vi "simulation.vi"() -> ()   [LabVIEW 2014]
uses:
  <vilib>/addons/Modulation/Digital/Support/Controls/Pack Bits Parameters.ctl
  <vilib>/addons/Modulation/Digital/General/MT Generate Bits (Galois, PN Order).vi
  <vilib>/addons/Modulation/Analog/support/mod_Set Error Source.vi
  <vilib>/addons/Modulation/Digital/Support/Common/Validators/mod_Generate Bits Validate.vi
  <vilib>/addons/Modulation/Digital/Support/Common/Validators/mod_AWGN Validate.vi
  <vilib>/addons/Modulation/Digital/Impairments/subVIs/mod_createSeeds.vi
  <vilib>/addons/Modulation/Digital/Support/Common/Validators/mod_Validate Samples Per Symbol.vi
  <vilib>/addons/Modulation/Analog/support/Validators/mod_Validate Complex Waveform.vi
  <vilib>/addons/Modulation/Analog/support/Validators/mod_WFErrorHandler.vi
  <vilib>/addons/Modulation/Digital/Support/Common/Validators/mod_Generate Filter Coefficients Validate.vi
  <vilib>/addons/Modulation/Digital/General/subVIs/mod_Generate Filter Coefficients.vi
  <vilib>/addons/Modulation/Digital/General/subVIs/mod_Generate Bits PN Sequence.vi
  <vilib>/addons/Modulation/Digital/General/MT Apply Pulse Shaping Filter (Generic).vi
  <vilib>/Analysis/1siggen.llb/Gaussian White Noise (obs 90).vi
  <vilib>/addons/Modulation/niDMT.lvlib
panel:
  out "XY Graph 2":cdb[](graph)
  in  "lpbw":dbl
  in  "nfilts":i32
  in  "noise density (dBc/Hz)":dbl=-120.0 format="%.2p"
  in  "Eb/N0 (10 dB)":dbl=10.0 format="%.2f"
  in  "bits per symbol (1)":i32=1
  out "decoded":i32
  out "iterations":i32
  out "bytes cluster":cluster{string}[](array[cluster])
  in  "type":enum16{"binary", "quadrature"}(ring)
  out "XY Graph":cdb[](graph)
  in  "total bits (128)":i32=128
  in  "stop":bool
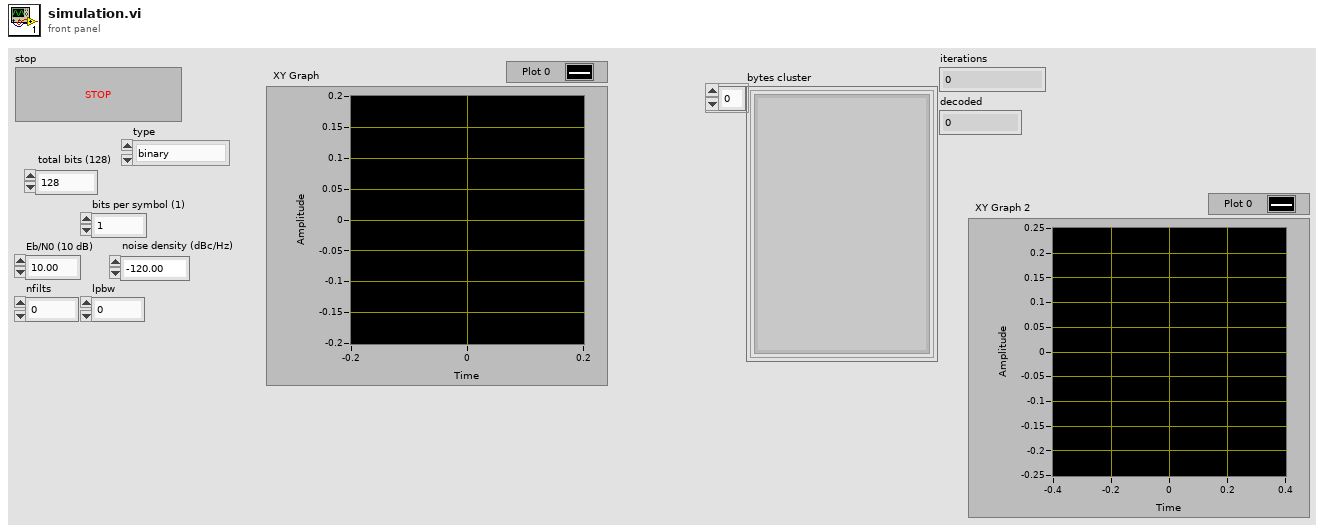
[diagram p1: front panel]
types:
  T1 = enum16{"none", "Raised Cosine", "Root Raised Cos", "Gaussian"}
  T2 = enum16{"FSK", "PSK", "QAM", "MSK", "PAM", "ASK", "CPM"}
  T3 = typedef "niDMT.lvlib/Pack Bits Parameters.ctl" = enum16{"Unsigned", "Signed"}
  T4 = typedef "niAMT.lvlib/Complex Data Waveform.ctl" = cluster{"t0":dbl, "dt":dbl, "Y":cdb[]}
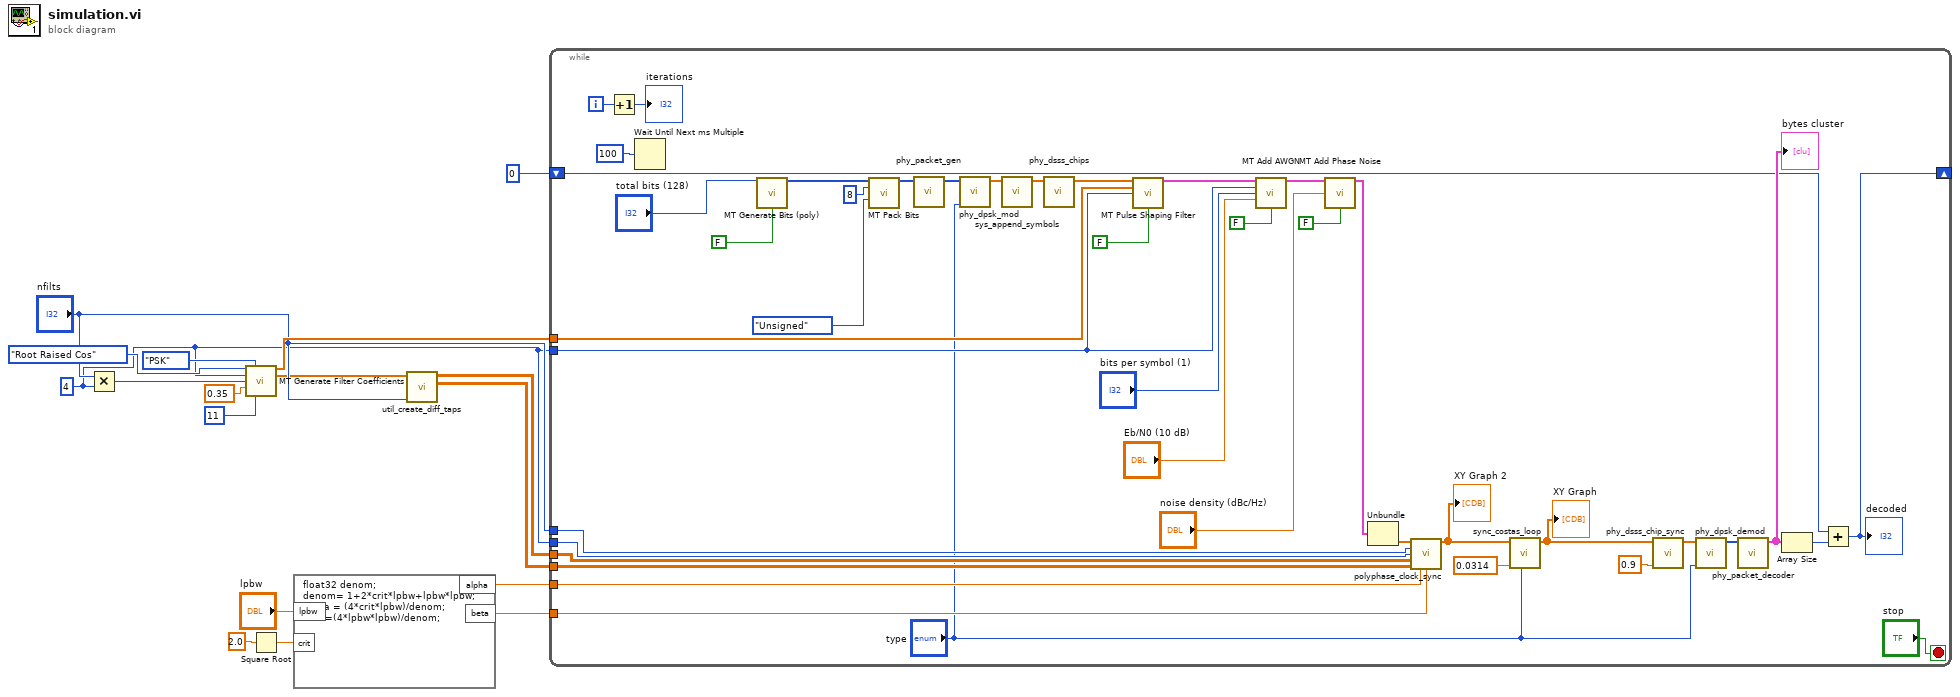
[diagram p0: block diagram]
diagram:
  w8 = 4 ("pulse shaping samples per symbol (16)")
  n1 = Multiply(x="nfilts", y=w8) -> (x*y=w1:i32)
  n2 = call <vilib>:"MT Generate Filter Coefficients.vi"("pulse shaping filter (none)"=T1."Root Raised Cos", "modulation type"=T2."PSK", "pulse shaping samples per symbol (16)"=w8, "matched samples per symbol (16)"=w1, "filter parameter"=0.35, "filter length (symbols)"=11) -> ("pulse shaping filter coefficients"=w12:dbl[], "matched filter coefficients"=w2:dbl[])  [unwired: 7 in, 1 out]
  n3 = Square Root(x=2.0) -> (sqrt(x)=w5:dbl)
  n4 = formula code="float32 denom; \ndenom= 1+2*crit*lpbw+lpbw*lpbw;\nalpha = (4*crit*lpbw)/denom;\nbeta=(4*lpbw*lpbw)/denom;"("lpbw"="lpbw", "crit"=w5) -> ("alpha"=w4:dbl, "beta"=w3:dbl)
  n5 = call "util_create_diff_taps.vi"("nfilts"="nfilts", "taps"=w2) -> ("out diff taps"=w10:dbl[][], "out taps"=w11:dbl[][])  [unwired: 7 in, 1 out]
  n6 = while {
    shift-right: [w43] -> _
    shift-left: 0 -> [w44]
    tunnel: w12 -> [w39]
    tunnel: w8 -> [w37]
    tunnel: w11 -> [w31]
    tunnel: w10 -> [w30]
    tunnel: "nfilts" -> [w29]
    tunnel: w8 -> [w28]
    tunnel: w4 -> [w27]
    tunnel: w3 -> [w26]
    i -> [w42]
    stop <- "stop" stop-if-true
    n7 = Increment(x=w42) -> (x+1=→"iterations":i32)
    n8 = Wait Until Next ms Multiple(millisecond multiple=u32 100) -> ()  [unwired: 1 out]
    n9 = call-poly <vilib>:"MT Generate Bits (poly).vi"("total bits (128)"="total bits (128)", "reset? (T)"=FALSE) -> ("output bit stream"=w55:i8[])  [unwired: 11 in, 2 out]
    n10 = call <vilib>:"MT Pack Bits.vi"("input bit stream"=w55, "bits per integer"=8, "integer format"=Pack_Bits_Parameters."Unsigned") -> ("output integers"=w52:i32[])  [unwired: 11 in, 1 out]
    n11 = call "phy_packet_gen.vi"("Input bytes"=w52) -> ("output bit stream"=w58:i8[])  [unwired: 10 in]
    n12 = call "phy_dpsk_mod.vi"("type"="type", "input bits"=w58) -> ("dpsk"=w57:cdb[])  [unwired: 8 in, 1 out]
    n13 = call "sys_append_symbols.vi"("raw symbols"=w57) -> ("appended symbols"=w56:cdb[])  [unwired: 10 in]
    n14 = call "phy_dsss_chips.vi"("symbols"=w56) -> ("chips"=w40:cdb[])  [unwired: 10 in]
    n15 = call-poly <vilib>:"MT Pulse Shaping Filter.vi"("symbols"=w40, "pulse shaping filter coefficients"=w39, "samples per symbol (16)"=w37, "reset? (T)"=FALSE) -> ("output complex waveform"=w38:T4)  [unwired: 10 in, 1 out]
    n16 = call <vilib>:"MT Add AWGN.vi"("input complex waveform"=w38, "samples per symbol (16)"=w37, "bits per symbol (1)"="bits per symbol (1)", "Eb/N0 (10 dB)"="Eb/N0 (10 dB)", "reset? (T)"=FALSE) -> ("output complex waveform"=w20:T4)  [unwired: 8 in, 2 out]
    n17 = call <vilib>:"MT Add Phase Noise.vi"("input complex waveform"=w20, "noise density (dBc/Hz)"="noise density (dBc/Hz)", "reset? (T)"=FALSE) -> ("output complex waveform"=w18:T4)  [unwired: 10 in, 2 out]
    n18 = Unbundle(w18) -> ("Y"=w22:cdb[])  [unwired: 2 out]
    n19 = call "polyphase_clock_sync.vi"("samples"=w22, "nfilts"=w29, "sps"=w28, "taps"=w31, "diff taps"=w30, "alpha"=w27, "beta"=w26) -> ("out symbols"=w21:cdb[])  [unwired: 7 in, 1 out]
    "XY Graph 2" <- w21
    n20 = call "sync_costas_loop.vi"("arity"="type", "loop bandwidth"=0.0314, "symbols"=w21) -> ("outputs"=w23:cdb[])  [unwired: 8 in]
    "XY Graph" <- w23
    n21 = call "phy_dsss_chip_sync.vi"("Threshold"=0.9, "dsss_chips"=w23) -> ("symbols"=w48:cdb[])  [unwired: 9 in]
    n22 = call "phy_dpsk_demod.vi"("arity"="type", "dpsk"=w48) -> ("bitstream"=w47:u8[])  [unwired: 9 in]
    n23 = call "phy_packet_decoder.vi"("bits"=w47) -> ("bytes cluster"=w46:cluster{string}[])  [unwired: 10 in]
    "bytes cluster" <- w46
    n24 = Array Size(array=w46) -> (size(s)=w45:i32)
    n25 = Add(x=w44, y=w45) -> (x+y=w43:i32)
    "decoded" <- w43
  }
